vi "CMD StartLog.vi"(8 "error in (no error)":errorcluster, 10 "TDMS File Name":string, 11 "Log_Engine in":refnum<class "Log_Engine.lvclass">) -> (0 "error out":errorcluster, 3 "Log_Engine out":refnum<class "Log_Engine.lvclass">)   [LabVIEW 2019, in "Log_Engine.lvclass"]
doc: "Developed by Kevin Thompson\nkevin@thompsonengineering.net\n\nCopyright 2018\nThompson Engineering, LLC"
uses:
  Log_Engine.lvclass
  DataTypes/AsynCmd_Log_Engine--enum.ctl
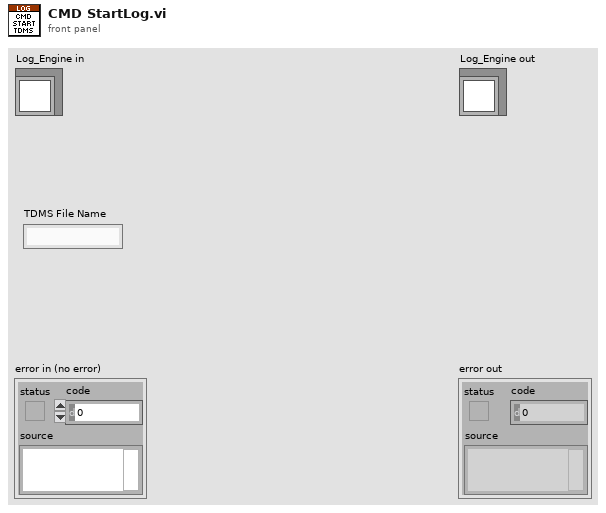
[diagram p1: front panel]
types:
  T1 = typedef "Log_Engine.lvclass/AsynCmd_Log_Engine--enum.ctl" = enum16{"Log_Engine.StartLog", "Log_Engine.StopLog", "Log_Engine.StartESRLog", "Log_Engine.StopESRLog"}
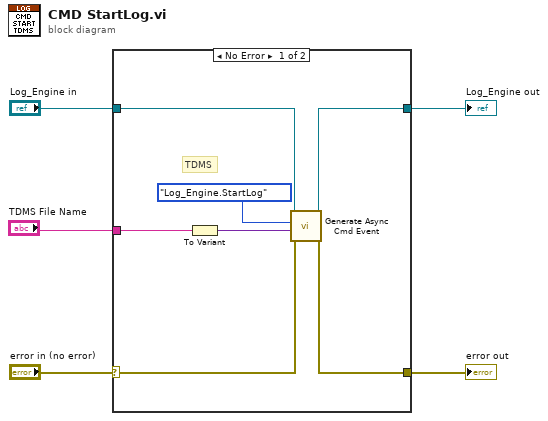
[diagram p0: block diagram]
diagram:
  n1 = case shown="No Error" "error in (no error)" {
    selector: "error in (no error)" -> [w10 w14]
    tunnel: [w9 w14] -> w4
    tunnel: [w11 w13] -> w2
    tunnel: "Log_Engine in" -> [w12 w13]
    tunnel: "TDMS File Name" -> [w7 _]
    frame No Error {
      # "TDMS"
      n2 = To Variant(anything=w7) -> (Variant=w6:variant)
      n3 = call "Generate Async Cmd Event.vi"("error in (no error)"=w10, "vData"=w6, "AsyncCmd"=AsynCmd_Log_Engine--enum."Log_Engine.StartLog", "Log_Engine in"=w12) -> ("error out"=w9:errorcluster, "Log_Engine out"=w11:refnum<class "Log_Engine.lvclass">)  [unwired: 6 in]
    }
    frame Error {
    }
  }
  "error out" <- w4
  "Log_Engine out" <- w2
